vi "下载图片AOI.vi"(8 "error in (no error)":errorcluster caption="错误输入（无错误）", 9 "文件类型":string(combo), 10 "产品型号":string="216") -> (0 "error out":errorcluster, 2 "获取成功":bool, 3 "文件路径":path[](array[path]), 7 "ServerResponseHead":string)   [LabVIEW 2014]
uses:
  <vilib>/Utility/NIReport.llb/NI_report.lvclass
  <vilib>/httpClient/LabVIEWHTTPClient.lvlib
panel:
  out "添加的路径":path
  out "ServerResponseBody_ANSI":string
  out "resulting string":string
  out "ServerResponseBody_UTF8":string
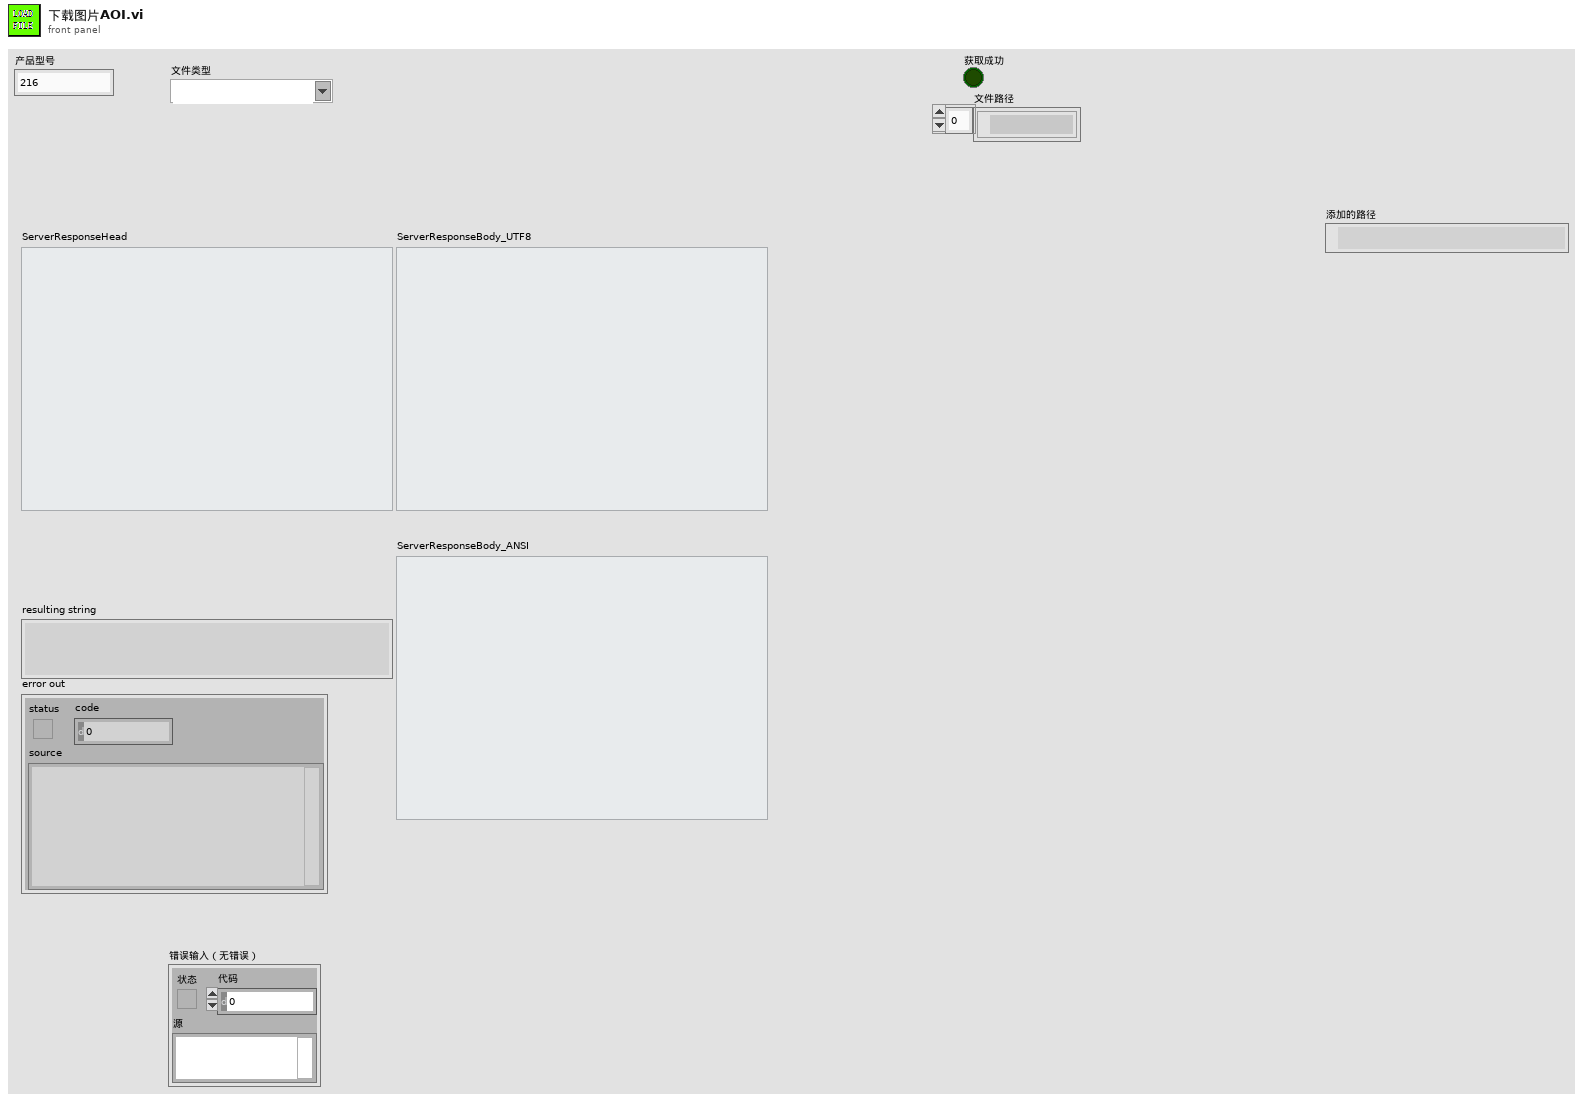
[diagram p1: front panel]
types:
  T1 = enum16{"Standard Report", "HTML", "Word", "Excel"}
  T2 = enum16{"maximized", "minimized", "normal", "no change"}
  T3 = typedef "LabVIEWHTTPClient.lvlib/ClientHandle.ctl" = refnum<k1>
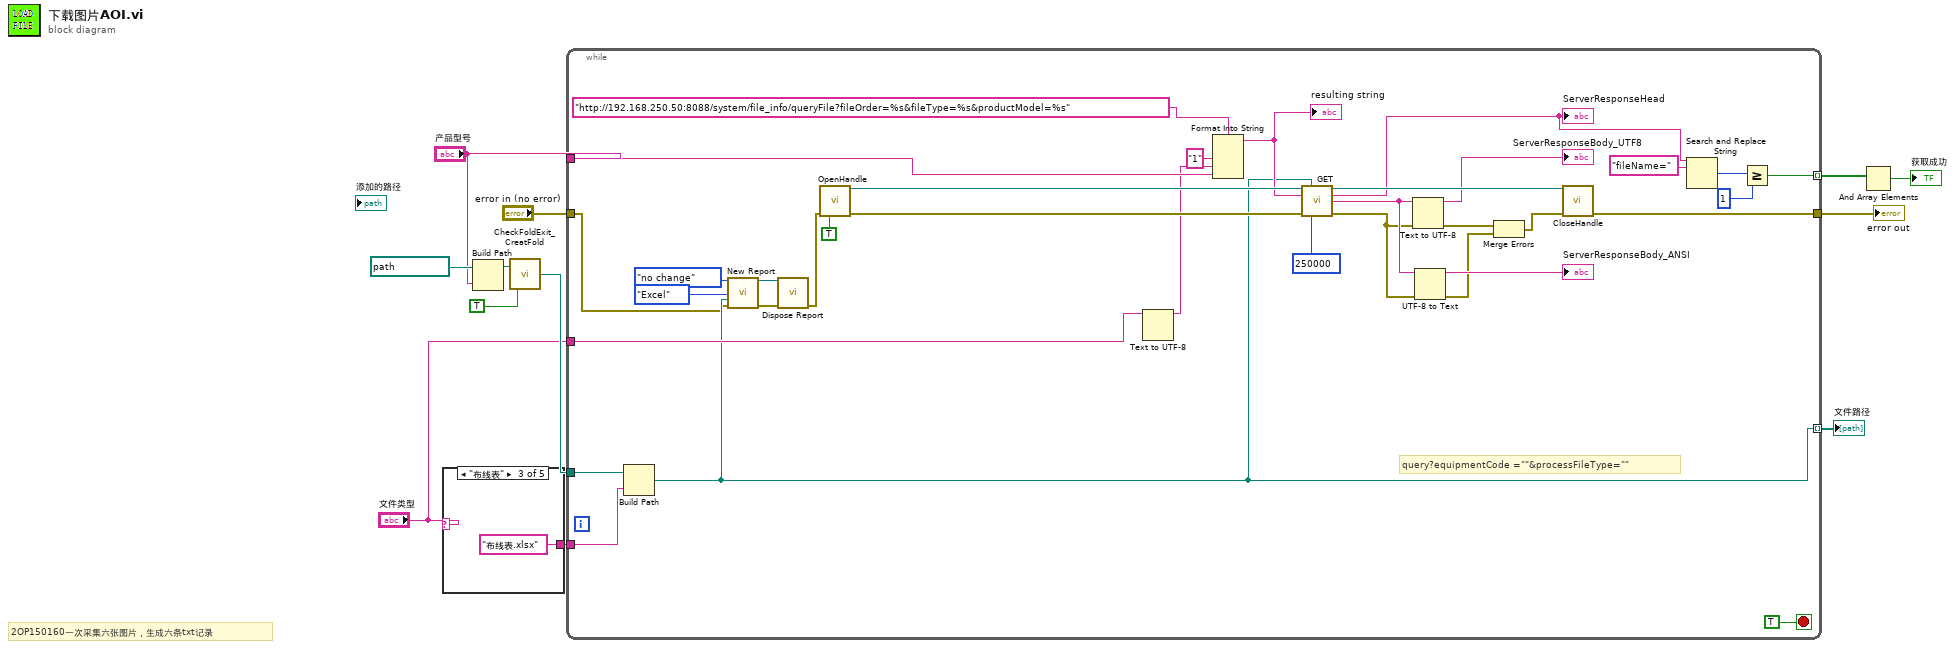
[diagram p0: block diagram]
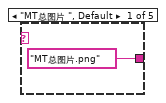
[diagram p2: hidden frame]
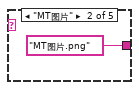
[diagram p3: hidden frame]
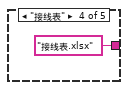
[diagram p4: hidden frame]
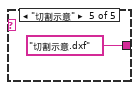
[diagram p5: hidden frame]
diagram:
  # "2OP150160一次采集六张图片，生成六条txt记录"
  n1 = case shown="\"布线表\"" "文件类型" {
    tunnel: ["MT总图片.png" ("字符串") "MT图片.png" ("字符串") "布线表.xlsx" ("字符串") "接线表.xlsx" ("字符串") "切割示意.dxf" ("字符串")] -> w5
    frame "MT总图片 ", Default {
    }
    frame "MT图片" {
    }
    frame "布线表" {
    }
    frame "接线表" {
    }
    frame "切割示意" {
    }
  }
  n2 = Build Path(base path=path "D:/临时文件" ("path in"), name or relative path="产品型号") -> (appended path=w1:path)
  n3 = call "CheckFoldExit_CreatFold.vi"("path in"=w1, "FoldOrFile¡H"=TRUE) -> ("Fold out"=w9:path)  [unwired: 2 out]
  n4 = while {
    tunnel: "error in (no error)" -> [w18]
    tunnel: [w40] -> w11
    tunnel: "产品型号" -> [w27]
    tunnel: [w33] -> w8 mode=indexing
    tunnel: w9 -> [w32]
    tunnel: [w20] -> w6 mode=indexing
    tunnel: w5 -> [w30]
    tunnel: "文件类型" -> [w29]
    stop <- TRUE stop-if-true
    # "query?equipmentCode =\"\"&processFileType=\"\""
    n5 = Build Path(base path=w32, name or relative path=w30) -> (appended path=w20:path)
    n6 = call <vilib>:"New Report.vi"("window state (normal)"=T2."no change", "report type"=T1."Excel", "template (empty)"=w20, "error in (no error)"=w18) -> ("report out"=w22:refnum<class "NI_report.lvclass">, "error out"=w21:errorcluster)  [unwired: 10 in]
    n7 = call-dynamic "Dispose Report.vi"("report in"=w22, "error in (no error)"=w21) -> ("error out"=w19:errorcluster)  [unwired: 13 in]
    n8 = call <vilib>:"OpenHandle.vi"("error in (no error)"=w19, "verify server(true)"=TRUE) -> ("client handle out"=w51:T3, "error out"=w50:errorcluster)  [unwired: 12 in]
    n9 = Text to UTF-8(11:w29) -> (3:w26:string)  [unwired: 2 in, 1 out]
    n10 = Format Into String(format string="http://192.168.250.50:8088/system/file_info/queryFile?fileOrder=%s&fileType=%s&productModel=%s" ("url"), "1" ("输入 1"), w26, w27) -> (resulting string=w38:string)  [unwired: 2 in, 1 out]
    "resulting string" <- w38
    n11 = call <vilib>:"GET.vi"("client handle"=w51, "output file"=w20, "url"=w38, "error in (no error)"=w50, "timeout (10000)"=250000) -> ("client handle out"=w49:T3, "headers"=w34:string, "body"=w45:string, "error out"=w44:errorcluster)  [unwired: 7 in]
    "ServerResponseHead" <- w34
    n12 = Text to UTF-8(8:w44, 11:w45) -> (0:w42:errorcluster, 3:→"ServerResponseBody_UTF8":string)  [unwired: 1 in]
    n13 = UTF-8 to Text(8:w44, 11:w45) -> (0:w39:errorcluster, 3:→"ServerResponseBody_ANSI":string)  [unwired: 1 in]
    n14 = Merge Errors(w42, w39) -> (w41:errorcluster)
    n15 = call <vilib>:"CloseHandle.vi"("client handle"=w49, "error in (no error)"=w41) -> ("error out"=w40:errorcluster)  [unwired: 13 in]
    n16 = Search and Replace String(input string=w34, search string="fileName=" ("搜索字符串")) -> (number of replacements=w36:i32)  [unwired: 6 in, 3 out]
    n17 = Greater Or Equal?(x=w36, y=1) -> (x >= y?=w33:bool)
  }
  "error out" <- w11
  "文件路径" <- w6
  n18 = And Array Elements(Boolean array=w8) -> (logical AND=→"获取成功":bool)
